vi "build_commands_T2.vi"(8 "Refocus_s":dbl, 9 "Refocus?":bool, 11 "T2_parameters":T1) -> (3 "Array out":T2(array[cluster]))   [LabVIEW 2014]
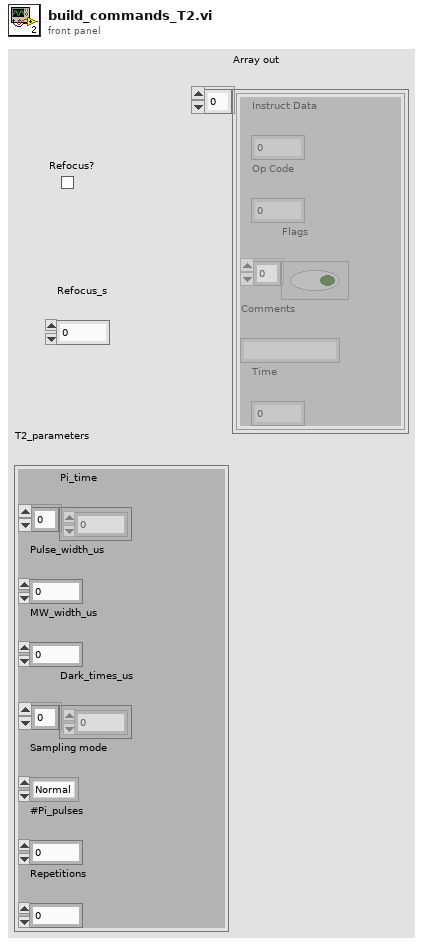
[diagram p1: front panel]
types:
  T1 = cluster{"Pi_time":dbl[], "Pulse_width_us":dbl, "MW_width_us":dbl, "Dark_times_us":dbl[], "Sampling mode":enum16{"Normal", "Sweep"}, "#Pi_pulses":i32, "Repetitions":i32}
  T2 = cluster{"Instruct Data":i32, "Op Code":i32, "Flags":bool[], "Comments":string, "Time":dbl}[]
  T3 = cluster{"Instruct Data":i32, "Op Code":i32, "Flags":bool[], "Comments":string, "Time":dbl}
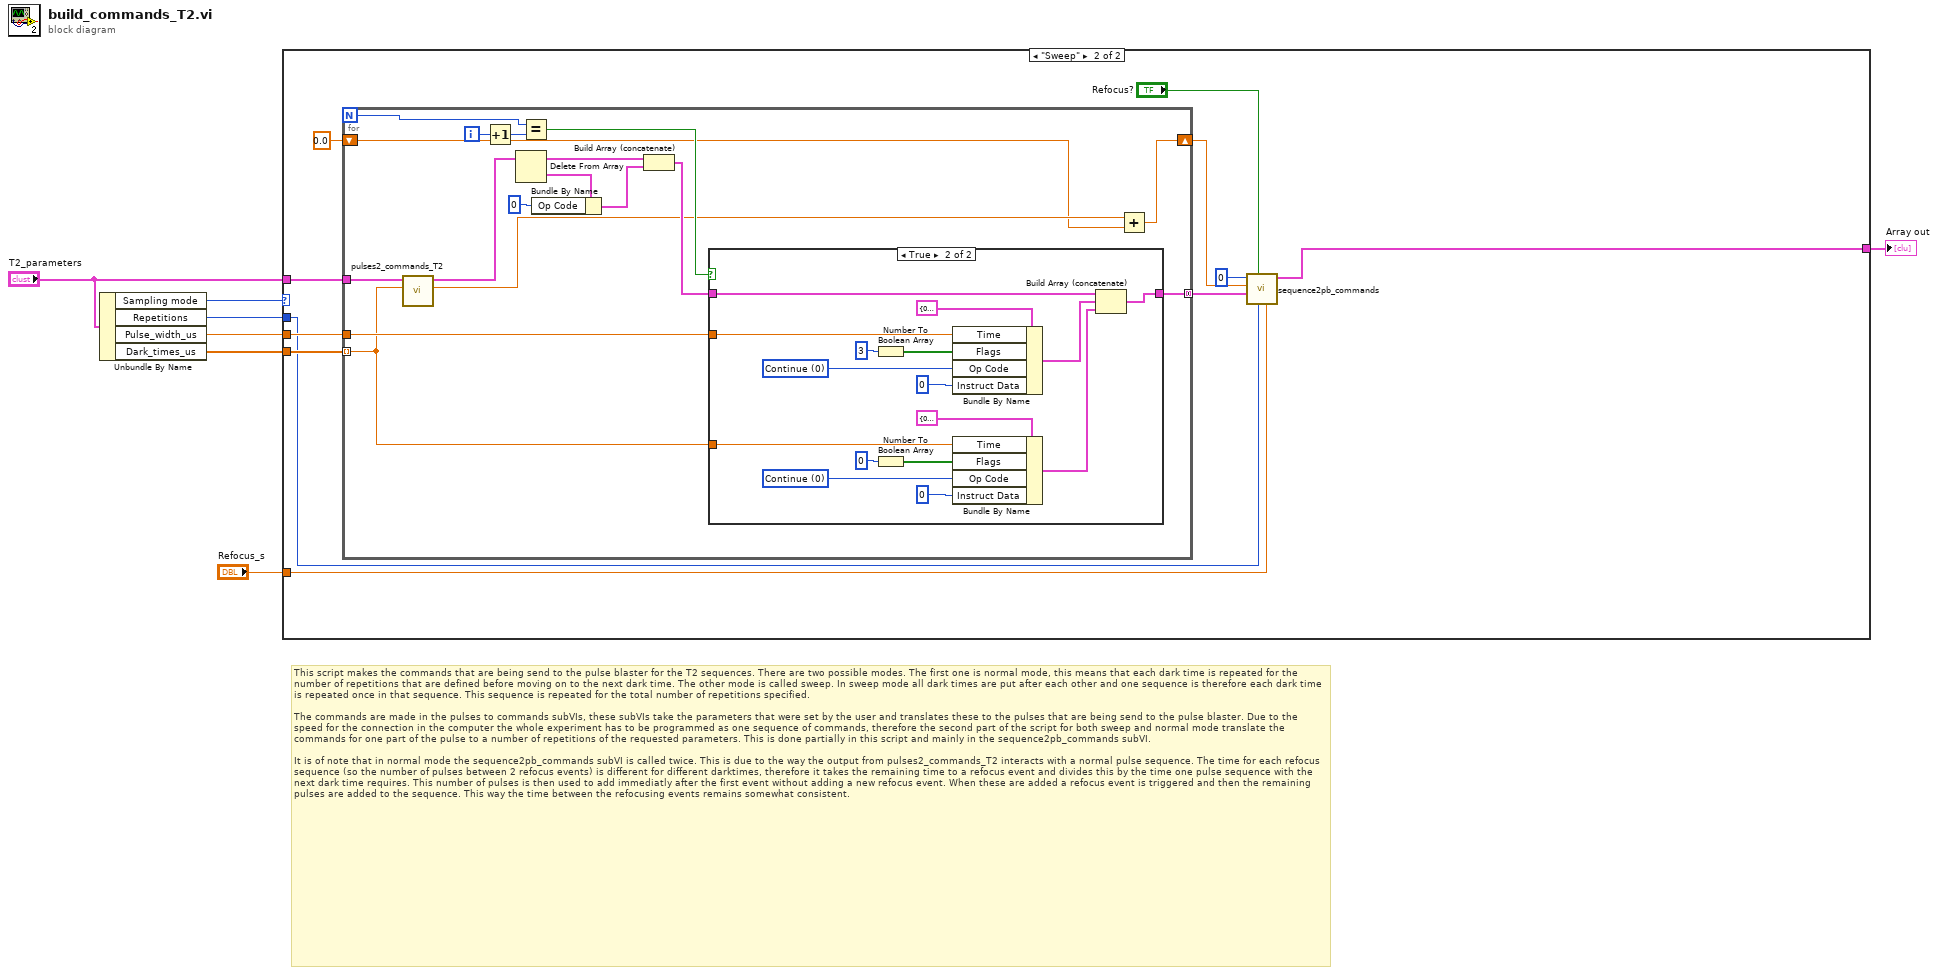
[diagram p0: block diagram]
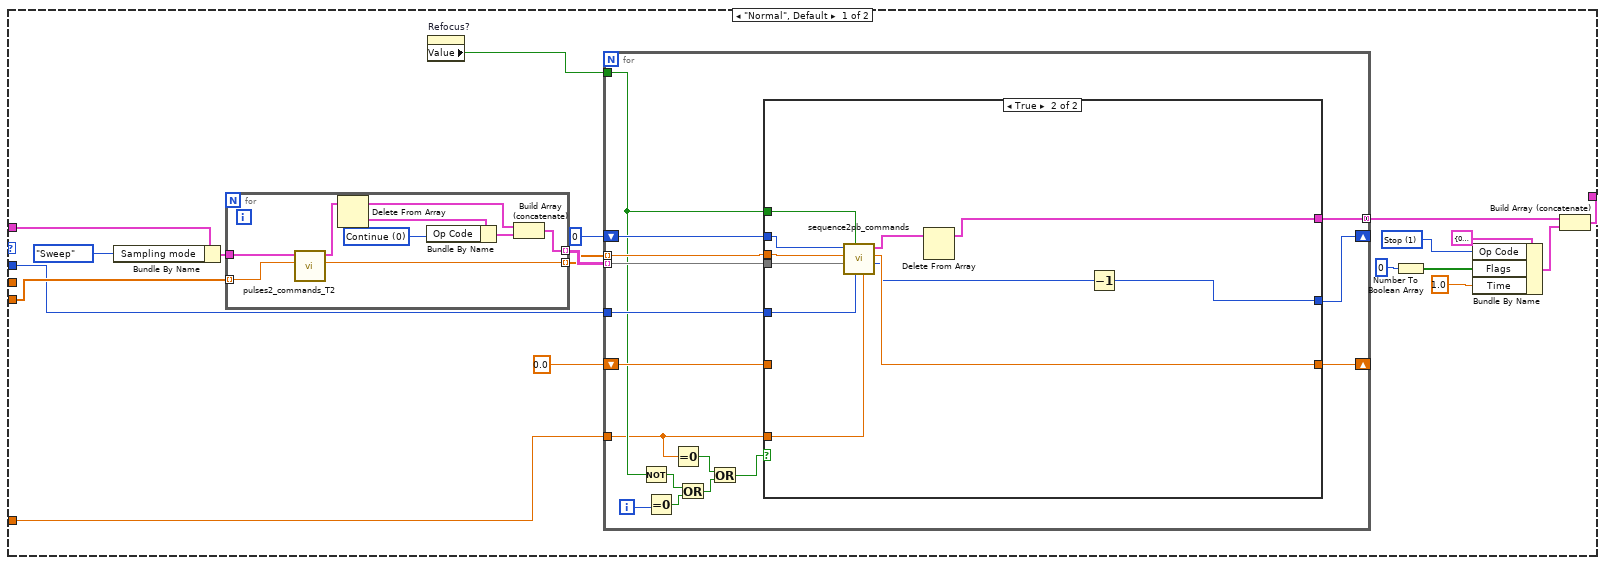
[diagram p2: hidden frame]
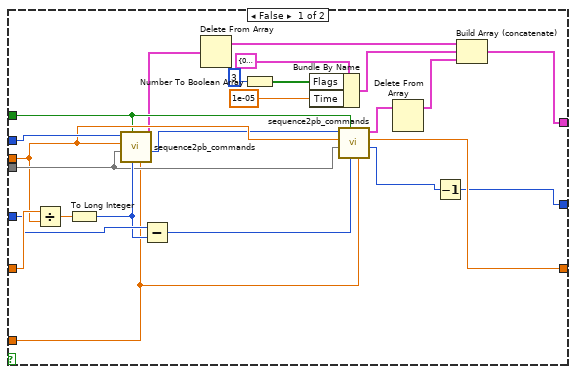
[diagram p3: hidden frame]
diagram:
  # "This script makes the commands that are being send to the pulse blaster for the T2 sequences. There are two possible modes. The first one is normal mode, this means that each dark time is repeated for the number of repetitions that are defined before moving on to the next dark time. The other mode is called sweep. In sweep mode all dark times are put after each other and one sequence is therefore each dark time is repeated once in that sequence. This sequence is repeated for the total number of repetitions specified.\n\nThe commands are made in the pulses to commands subVIs, these subVIs take the parameters that were set by the user and translates these to the pulses that are being send to the pulse blaster. Due to the speed for the connection in the computer the whole experiment has to be programmed as one sequence of commands, therefore the second part of the script for both sweep and normal mode translate the commands for one part of the pulse to a number of repetitions of the requested parameters. This is done partially in this script and mainly in the sequence2pb_commands subVI.\n\nIt is of note that in normal mode the sequence2pb_commands subVI is called twice. This is due to the way the output from pulses2_commands_T2 interacts with a normal pulse sequence. The time for each refocus sequence (so the number of pulses between 2 refocus events) is different for different darktimes, therefore it takes the remaining time to a refocus event and divides this by the time one pulse sequence with the next dark time requires. This number of pulses is then used to add immediatly after the first event without adding a new refocus event. When these are added a refocus event is triggered and then the remaining pulses are added to the sequence. This way the time between the refocusing events remains somewhat consistent."
  n1 = Unbundle By Name("T2_parameters") -> ("Sampling mode"=w7:enum16{"Normal", "Sweep"}, "Repetitions"=w3:i32, "Pulse_width_us"=w2:dbl, "Dark_times_us"=w1:dbl[])
  n2 = case shown="\"Sweep\"" w7 {
    tunnel: "Refocus_s" -> [w9 w91]
    tunnel: w3 -> [w8 w89]
    tunnel: "T2_parameters" -> [w26 w97]
    tunnel: [w17 w87] -> w4
    tunnel: w2 -> [_ w93]
    tunnel: w1 -> [w23 w92]
    frame "Normal", Default {
      w13 = 1 items=["Continue", "Stop", "Loop", "End Loop", "JSR", "RTS", "Branch", "Long Delay", "Wait"] ("Op Code 2")
      n3 = Bundle By Name(cluster=w26, "Sampling mode"=enum16{"Normal", "Sweep"}."Sweep") -> (w24:T1)
      n4 = for {
        tunnel: w24 -> [w86]
        tunnel: w23 -> [w84] mode=indexing
        tunnel: [w83] -> w22 mode=indexing
        tunnel: [w85] -> w21 mode=indexing
        w81 = 0 items=["Continue", "Stop", "Loop", "End Loop", "JSR", "RTS", "Branch", "Long Delay", "Wait"] ("Op Code 2")
        n5 = call "pulses2_commands_T2.vi"("Dark_time_us"=w84, "T2_parameters"=w86) -> ("Sequence_time_us"=w85:dbl, "Array out"=w79:T2)  [unwired: 8 in]
        n6 = Delete From Array(array=w79) -> (deleted portion=w82:T3, array with subset deleted=w78:T2)  [unwired: 2 in]
        n7 = Bundle By Name(cluster=w82, "Op Code"=w81) -> (w80:T3)
        n8 = Build Array (concatenate)(w78, w80) -> (w83:T2)
      }
      n9 = property on="Refocus?" class="Bool (strict)"() -> ("Value"=w19:bool)  [unwired: 2 in, 2 out]
      n10 = for {
        tunnel: w22 -> [w41] mode=indexing
        tunnel: w21 -> [w40] mode=indexing
        tunnel: w19 -> [w33]
        shift-right: [w36] -> _
        shift-left: 0 -> [w39]
        tunnel: w9 -> [w29]
        tunnel: w8 -> [w42]
        shift-right: [w37] -> _
        shift-left: 0.0 -> [w38]
        tunnel: [w27] -> w11 mode=concatenating
        i -> [w35]
        n11 = Not(x=w33) -> (.not. x?=w32:bool)
        n12 = Equal To 0?(x=w35) -> (x = 0?=w34:bool)
        n13 = Equal To 0?(x=w29) -> (x = 0?=w30:bool)
        n14 = Or(x=w32, y=w34) -> (x .or. y?=w31:bool)
        n15 = Or(x=w30, y=w31) -> (x .or. y?=w28:bool)
        n16 = case shown="True" w28 {
          tunnel: w29 -> [w57 w77]
          tunnel: w42 -> [w64 w76]
          tunnel: w41 -> [w60 w75]
          tunnel: w40 -> [w59 w74]
          tunnel: w39 -> [w61 w73]
          tunnel: w33 -> [w58 w72]
          tunnel: w38 -> [w66 _]
          tunnel: [w56 w70] -> w37
          tunnel: [w50 w68] -> w36
          tunnel: [w52 w67] -> w27
          frame False {
            n17 = Divide(x=w66, y=w59) -> (x/y=w65:dbl)
            n18 = To Long Integer(number=w65) -> (32bit integer=w63:i32)
            n19 = call "sequence2pb_commands.vi"("Refocus_s"=w57, "Repetitions"=w63, "Refocus?"=w58, "command_sequence"=w60, "Sequence_length"=w59, "start_command"=w61) -> ("end_command"=w43:i32, "PB_commands"=w54:T2)  [unwired: 3 in, 1 out]
            n20 = Subtract(x=w64, y=w63) -> (x-y=w62:i32)
            n21 = Delete From Array(array=w54) -> (array with subset deleted=w53:T2)  [unwired: 2 in, 1 out]
            n22 = Number To Boolean Array(number=3) -> (Boolean array=w47:bool[])
            n23 = Bundle By Name(cluster=T3 {"Instruct Data"=0, "Op Code"=0, "Flags"=[FALSE, FALSE, FALSE, FALSE, FALSE, FALSE, FALSE, FALSE, FALSE, FALSE, FALSE, FALSE, FALSE, FALSE, FALSE, FALSE, FALSE, FALSE, FALSE, FALSE, FALSE, FALSE, FALSE, FALSE], "Comments"="", "Time"=1e-06} ("PB Instruction"), "Flags"=w47, "Time"=1e-05) -> (w44:T3)
            n24 = call "sequence2pb_commands.vi"("Refocus_s"=w57, "Repetitions"=w62, "Refocus?"=w58, "command_sequence"=w60, "Sequence_length"=w59, "start_command"=w43) -> ("end_command"=w51:i32, "t_remaining"=w56:dbl, "PB_commands"=w55:T2)  [unwired: 3 in]
            n25 = Delete From Array(array=w55) -> (array with subset deleted=w49:T2)  [unwired: 2 in, 1 out]
            n26 = Decrement(x=w51) -> (x-1=w50:i32)
            n27 = Build Array (concatenate)(w53, w44, w49) -> (w52:T2)
          }
          frame True {
            n28 = call "sequence2pb_commands.vi"("Refocus_s"=w77, "Repetitions"=w76, "Refocus?"=w72, "command_sequence"=w75, "Sequence_length"=w74, "start_command"=w73) -> ("end_command"=w69:i32, "t_remaining"=w70:dbl, "PB_commands"=w71:T2)  [unwired: 3 in]
            n29 = Delete From Array(array=w71) -> (array with subset deleted=w67:T2)  [unwired: 2 in, 1 out]
            n30 = Decrement(x=w69) -> (x-1=w68:i32)
          }
        }
      }
      n31 = Number To Boolean Array(number=0) -> (Boolean array=w15:bool[])
      n32 = Bundle By Name(cluster=T3 {"Instruct Data"=0, "Op Code"=0, "Flags"=[FALSE, FALSE, FALSE, FALSE, FALSE, FALSE, FALSE, FALSE, FALSE, FALSE, FALSE, FALSE, FALSE, FALSE, FALSE, FALSE, FALSE, FALSE, FALSE, FALSE, FALSE, FALSE, FALSE, FALSE], "Comments"="", "Time"=1e-06} ("PB Instruction"), "Op Code"=w13, "Flags"=w15, "Time"=1.0) -> (w10:T3)
      n33 = Build Array (concatenate)(w11, w10) -> (w17:T2)
    }
    frame "Sweep" {
      n34 = for {
        N -> [w112]
        tunnel: [w105] -> w94 mode=concatenating
        tunnel: w97 -> [w104]
        shift-right: [w101] -> w95
        shift-left: 0.0 -> [w102]
        tunnel: w93 -> [w99]
        tunnel: w92 -> [w98] mode=indexing
        i -> [w114]
        n35 = call "pulses2_commands_T2.vi"("Dark_time_us"=w98, "T2_parameters"=w104) -> ("Sequence_time_us"=w103:dbl, "Array out"=w100:T2)  [unwired: 8 in]
        n36 = Increment(x=w114) -> (x+1=w113:i32)
        n37 = Delete From Array(array=w100) -> (deleted portion=w111:T3, array with subset deleted=w108:T2)  [unwired: 2 in]
        n38 = Equal?(x=w112, y=w113) -> (x = y?=w107:bool)
        n39 = Bundle By Name(cluster=w111, "Op Code"=0) -> (w109:T3)
        n40 = Build Array (concatenate)(w108, w109) -> (w106:T2)
        n41 = case shown="True" w107 {
          tunnel: w106 -> [w115 w131]
          tunnel: [w115 w130] -> w105
          tunnel: w98 -> [_ w118]
          tunnel: w99 -> [_ w116]
          frame False {
          }
          frame True {
            w122 = 0 items=["Continue", "Stop", "Loop", "End Loop", "JSR", "RTS", "Branch", "Long Delay", "Wait"] ("Op Code 2")
            w126 = 0 items=["Continue", "Stop", "Loop", "End Loop", "JSR", "RTS", "Branch", "Long Delay", "Wait"] ("Op Code 2")
            n42 = Number To Boolean Array(number=3) -> (Boolean array=w127:bool[])
            n43 = Number To Boolean Array(number=0) -> (Boolean array=w119:bool[])
            n44 = Bundle By Name(cluster=T3 {"Instruct Data"=0, "Op Code"=0, "Flags"=[FALSE, FALSE, FALSE, FALSE, FALSE, FALSE, FALSE, FALSE, FALSE, FALSE, FALSE, FALSE, FALSE, FALSE, FALSE, FALSE, FALSE, FALSE, FALSE, FALSE, FALSE, FALSE, FALSE, FALSE], "Comments"="", "Time"=1e-06} ("PB Instruction"), "Time"=w116, "Flags"=w127, "Op Code"=w126, "Instruct Data"=0) -> (w124:T3)
            n45 = Bundle By Name(cluster=T3 {"Instruct Data"=0, "Op Code"=0, "Flags"=[FALSE, FALSE, FALSE, FALSE, FALSE, FALSE, FALSE, FALSE, FALSE, FALSE, FALSE, FALSE, FALSE, FALSE, FALSE, FALSE, FALSE, FALSE, FALSE, FALSE, FALSE, FALSE, FALSE, FALSE], "Comments"="", "Time"=1e-06} ("PB Instruction"), "Time"=w118, "Flags"=w119, "Op Code"=w122, "Instruct Data"=0) -> (w117:T3)
            n46 = Build Array (concatenate)(w131, w124, w117) -> (w130:T2)
          }
        }
        n47 = Add(x=w103, y=w102) -> (x+y=w101:dbl)
      }
      n48 = call "sequence2pb_commands.vi"("Refocus_s"=w91, "Repetitions"=w89, "Refocus?"="Refocus?", "command_sequence"=w94, "Sequence_length"=w95, "start_command"=0) -> ("PB_commands"=w87:T2)  [unwired: 3 in, 2 out]
    }
  }
  "Array out" <- w4
